vi "include_libsvm.vi"   [LabVIEW 2014]
uses:
  bin/x64/libsvm.dll
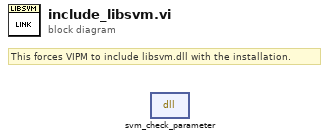
[diagram p0: block diagram]
diagram:
  # "This forces VIPM to include libsvm.dll with the installation."
  n1 = dll-call lib="C:/dev/LVLibSVM/LabVIEW/bin/x64/libsvm.dll" fn="svm_check_parameter"() -> ()  [unwired: 4 in, 2 out]
